vi "PrintBandwidthChart.vi"(7 "Path":path=path "C:/LabViewTesty", 9 "Colors 2":u32[](array[colorbox])=[11796480, 37103, 40712, 16770816, 11796658, 4210752], 10 "Bandwidth":string[](array[string]), 11 "Pie Chart Bandwidth of Frame":picture) -> ()   [LabVIEW 2014]
panel:
  out "Bandwidth":T1={"Pie Chart Bandwidth of Frame"=bytes[270], "Date"="", "Time"="", "Colors 2"=[11796480, 37103, 40712, 16770816, 11796658, 4210752], "Bandwidth"=[]}
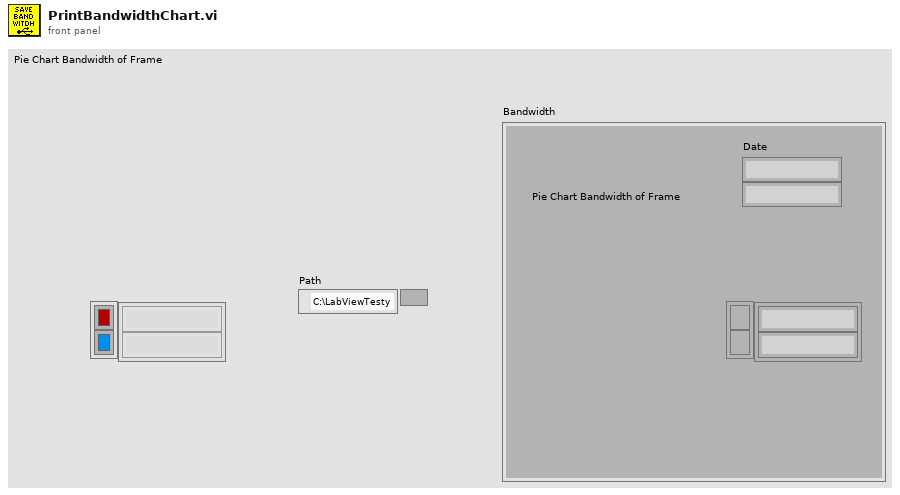
[diagram p1: front panel]
types:
  T1 = cluster{"Pie Chart Bandwidth of Frame":picture, "Date":string, "Time":string, "Colors 2":u32[], "Bandwidth":string[]}
  T2 = typedef "imagedata.ctl" = cluster{"image type":i32, "image depth":i32, "image":u8[], "mask":u8[], "colors":u32[], "Rectangle":cluster{"left":i16, "top":i16, "right":i16, "bottom":i16}}
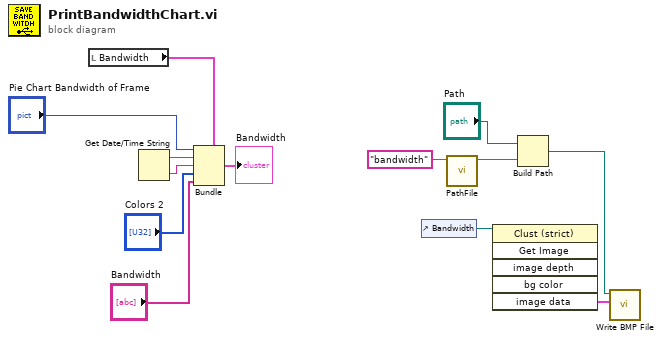
[diagram p0: block diagram]
diagram:
  n1 = local read "Bandwidth"() -> (w13:T1)
  n2 = Get Date/Time String() -> (date string=w9:string, time string=w8:string)  [unwired: 3 in]
  n3 = Bundle(cluster=w13, "Pie Chart Bandwidth of Frame"="Pie Chart Bandwidth of Frame", "Date"=w9, "Time"=w8, "Colors 2"="Colors 2", "Bandwidth"="Bandwidth") -> (→"Bandwidth":T1)
  n4 = control-ref of="Bandwidth"() -> (w1:refnum<vi>)
  n5 = call "PathFile.vi"("NameFile"="bandwidth") -> ("stringNameFile"=w2:string)  [unwired: 10 in]
  n6 = invoke class="Clust (strict)" method="Get Image"(reference=w1) -> ("image data"=w6:T2)  [unwired: 5 in, 5 out]
  n7 = Build Path(base path="Path", name or relative path=w2) -> (appended path=w5:path)
  n8 = call <vilib>:"Write BMP File.vi"("image data"=w6, "path to BMP file"=w5) -> ()  [unwired: 8 in, 2 out]
